vi "Store Data.vi"(8 "error in (no error)":errorcluster, 9 "Data":refnum<class "AbstractData.lvclass">, 10 "Name":string, 11 "StorageService in":refnum<class "StorageService.lvclass">) -> (0 "error out":errorcluster, 3 "StorageService out":refnum<class "StorageService.lvclass">)   [LabVIEW 2014, in "StorageService.lvclass"]
uses:
  StorageService.lvclass
  Model/Data/AbstractData/AbstractData.lvclass
  StorageService.lvclass/StorageService.ctl
  Interfaces/Observable Actor/Observable Actor.lvclass
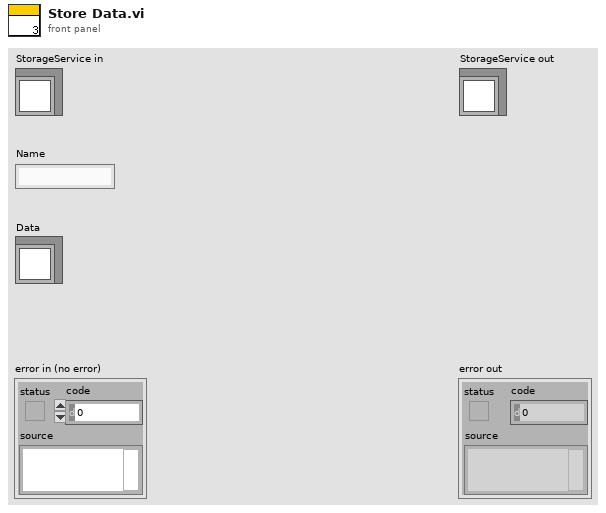
[diagram p1: front panel]
types:
  T1 = cluster{"Data":refnum<class "AbstractData.lvclass">, "Parameter":refnum<class "AbstractData.lvclass">}
  T2 = typedef "StorageService.lvclass/RegisteredObject.ctl" = cluster{"Name":string, "Is Acquired":bool, "Queue":refnum<queue>, "Message To Send":cluster{"Enqueuer":refnum<class "Message Enqueuer.lvclass">, "Message":refnum<class "ReplayData Msg.lvclass">}, "Save Parameters":variant}
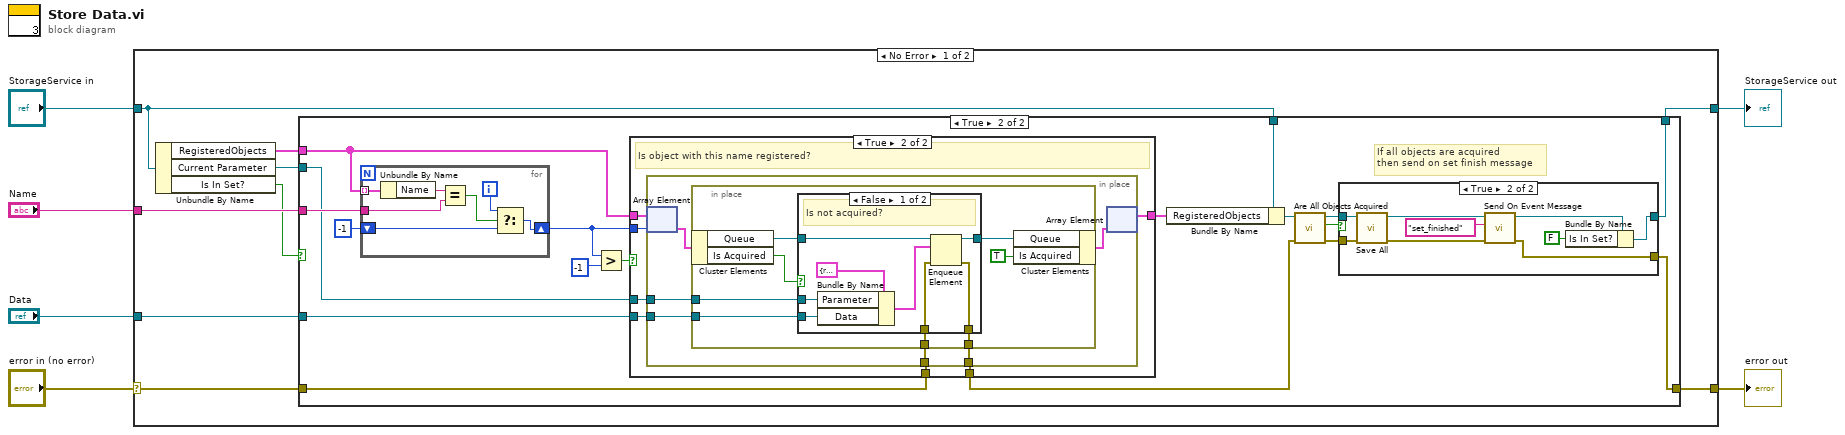
[diagram p0: block diagram]
diagram:
  n1 = case shown="No Error" "error in (no error)" {
    selector: "error in (no error)" -> [w12 w88]
    tunnel: [w11 w88] -> w5
    tunnel: [w7 w87] -> w3
    tunnel: "StorageService in" -> [w9 w87]
    tunnel: "Name" -> [w15 _]
    tunnel: "Data" -> [w13 _]
    frame No Error {
      n2 = Unbundle By Name(w9) -> ("RegisteredObjects"=w10:T2[], "Current Parameter"=w14:refnum<class "AbstractData.lvclass">, "Is In Set?"=w8:bool)
      n3 = case shown="True" w8 {
        tunnel: w15 -> [_ w35]
        tunnel: w14 -> [_ w33]
        tunnel: w13 -> [_ w32]
        tunnel: w12 -> [w17 w31]
        tunnel: [w17 w18] -> w11
        tunnel: w10 -> [_ w27]
        tunnel: w9 -> [w16 w25]
        tunnel: [w16 w20] -> w7
        frame False {
        }
        frame True {
          # "If all objects are acquired\nthen send on set finish message"
          n4 = for {
            tunnel: w27 -> [w86] mode=indexing
            tunnel: w35 -> [w85]
            shift-right: [w80] -> w29
            shift-left: -1 -> [w81]
            i -> [w82]
            n5 = Unbundle By Name(w86) -> ("Name"=w84:string)
            n6 = Equal?(x=w84, y=w85) -> (x = y?=w83:bool)
            n7 = Select(t=w82, s=w83, f=w81) -> (s? t:f=w80:i32)
          }
          n8 = Greater?(x=w29, y=-1) -> (0:w28:bool)
          n9 = case shown="True" w28 {
            tunnel: w33 -> [_ w55]
            tunnel: w32 -> [_ w54]
            tunnel: w31 -> [w48 w53]
            tunnel: [w48 w52] -> w19
            tunnel: w29 -> [_ w50]
            tunnel: w27 -> [w47 w51]
            tunnel: [w47 w49] -> w26
            frame False {
            }
            frame True {
              # "Is object with this name registered?"
              n10 = in-place {
                in-place-border: w55 -> [w61]
                in-place-border: w54 -> [w60]
                in-place-border: w53 -> [w59]
                in-place-border: [w58] -> w52
                n11 = in-place-array #1(w51, w50) -> (w57:T2)
                n12 = in-place {
                  in-place-border: w61 -> [w67]
                  in-place-border: w60 -> [w66]
                  in-place-border: w59 -> [w65]
                  in-place-border: [w64] -> w58
                  n13 = in-place-cluster #2(w57) -> ("Queue"=w69:refnum<queue>, "Is Acquired"=w62:bool)
                  n14 = case shown="False" w62 {
                    tunnel: w69 -> [w77 w78]
                    tunnel: w67 -> [w75 _]
                    tunnel: w66 -> [w74 _]
                    tunnel: w65 -> [w72 w79]
                    tunnel: [w71 w79] -> w64
                    tunnel: [w70 w78] -> w68
                    frame False {
                      # "Is not acquired?"
                      n15 = Bundle By Name(cluster=T1 {"Data"=refnum, "Parameter"=refnum} ("element"), "Parameter"=w75, "Data"=w74) -> (w73:T1)
                      n16 = Enqueue Element(queue=w77, element=w73, error in (no error)=w72) -> (queue out=w70:refnum<queue>, error out=w71:errorcluster)  [unwired: 1 in, 1 out]
                    }
                    frame True {
                    }
                  }
                  n17 = in-place-cluster #2("Queue"=w68, "Is Acquired"=TRUE) -> (w56:T2)
                }
                n18 = in-place-array #1(w56) -> (w49:T2[])  [unwired: 1 out]
              }
            }
          }
          n19 = Bundle By Name(cluster=w25, "RegisteredObjects"=w26) -> (w24:refnum<class "StorageService.lvclass">)
          n20 = call-dynamic "Are All Objects Acquired.vi"("error in (no error)"=w19, "StorageService in"=w24) -> ("error out"=w21:errorcluster, "All Is Acquired?"=w23:bool, "StorageService out"=w22:refnum<class "StorageService.lvclass">)  [unwired: 7 in]
          n21 = case shown="True" w23 {
            tunnel: w22 -> [w37 w45]
            tunnel: w21 -> [w36 w44]
            tunnel: [w37 w43] -> w20
            tunnel: [w36 w39] -> w18
            frame False {
            }
            frame True {
              n22 = call-dynamic "Save All.vi"("error in (no error)"=w44, "StorageService in"=w45) -> ("error out"=w40:errorcluster, "StorageService out"=w41:refnum<class "StorageService.lvclass">)  [unwired: 8 in]
              n23 = call "Send On Event Message.vi"("error in (no error)"=w40, "Event"="set_finished", "Observable Actor in"=w41) -> ("error out"=w39:errorcluster, "Observable Actor out"=w38:refnum<class "StorageService.lvclass">)  [unwired: 7 in]
              n24 = Bundle By Name(cluster=w38, "Is In Set?"=FALSE) -> (w43:refnum<class "StorageService.lvclass">)
            }
          }
        }
      }
    }
    frame Error {
    }
  }
  "error out" <- w5
  "StorageService out" <- w3
